vi "Lights and Music.vi"() -> ()   [LabVIEW 2013, in "LVH-Hue.lvlib"]
uses:
  LVH-Hue.lvlib
  <vilib>/sound2/lvsound2.llb/Sampling Mode.ctl
  Private/Type Defs/HSB.ctl
  <vilib>/sound2/lvsound2.llb/Sound File Info (path).vi
  <vilib>/sound2/lvsound2.llb/Sound File Read Open.vi
  <vilib>/sound2/lvsound2.llb/Sound File Read (DBL).vi
  <vilib>/measure/matone.llb/Extract Single Tone Information 1 Chan.vi
  Private/Set Light HSB By ID.vi
  <vilib>/sound2/lvsound2.llb/Sound Output Write (DBL Single).vi
  <vilib>/measure/NI_MAPro.lvlib
panel:
  in  "Hostname / IP":string="192.168.1.3"
  in  "Username":string="newdeveloper"
  in  "Lower Cut-Off":dbl=50.0
  out "Amp":dbl(graph)=0.00013614008667128265
  out "Freq":dbl(graph)=34.77410975578877
  out "detected frequency":dbl=34.77410975578877 format="%.2p"
  out "detected amplitude":dbl=0.00013614008667128265 format="%.2p"
  in  "Number of Samples/Iteration":i32=3500
  in  "Device ID":u32
  in  "Stop":bool
  out "Current Iteration":i32=32
  out "Raw Data":waveform(dbl)(graph)={"t0"=timestamp(1.8140589569160999 s since 1904-01-01), "dt"=2.2675736961451248e-05, "Y"=array[2500 elements]}
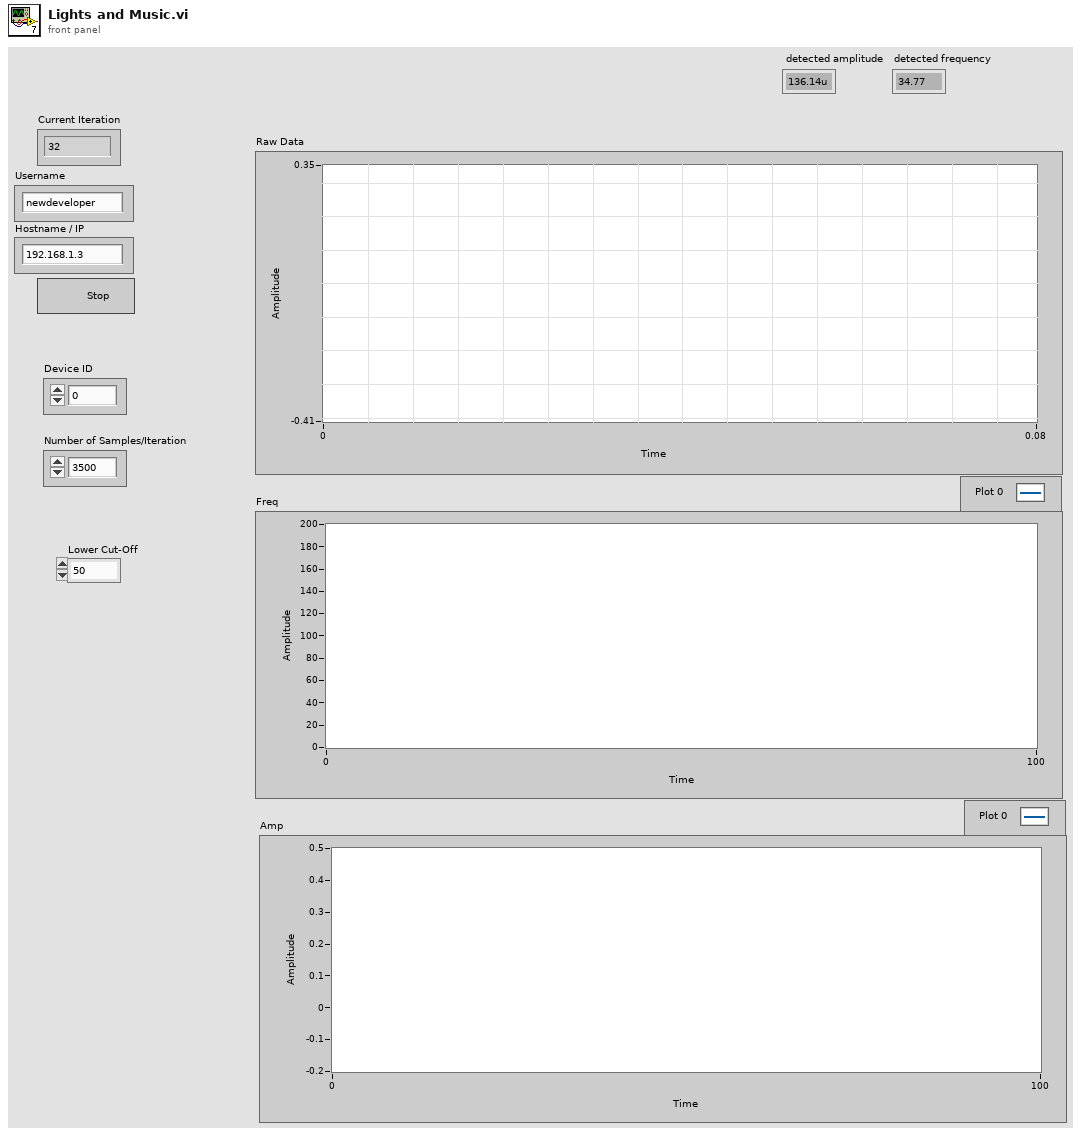
[diagram p1: front panel]
types:
  T1 = typedef "Sampling Mode.ctl" = i32
  T2 = typedef "Sound Data Format.ctl" = cluster{"sample rate (S/s)":dbl, "number of channels":i32, "bits per sample":i32}
  T3 = typedef "Sound File Refnum.ctl" = refnum<file>
  T4 = typedef "LVH-Hue.lvlib/Hue Ref.ctl" = cluster{"HTTP Session":T5, "Base URL":string, "Lights":T6[]}
  T5 = typedef "LabVIEWHTTPClient.lvlib/ClientHandle.ctl" = refnum<k1>
  T6 = typedef "LVH-Hue.lvlib/Light.ctl" = cluster{"ID":i32, "Name":string}
  T7 = typedef "Sound Output Task ID.ctl" = u32
  T8 = typedef "LVH-Hue.lvlib/HSB.ctl" = cluster{"Hue":u16, "Saturation":u8, "Brightness":u8}
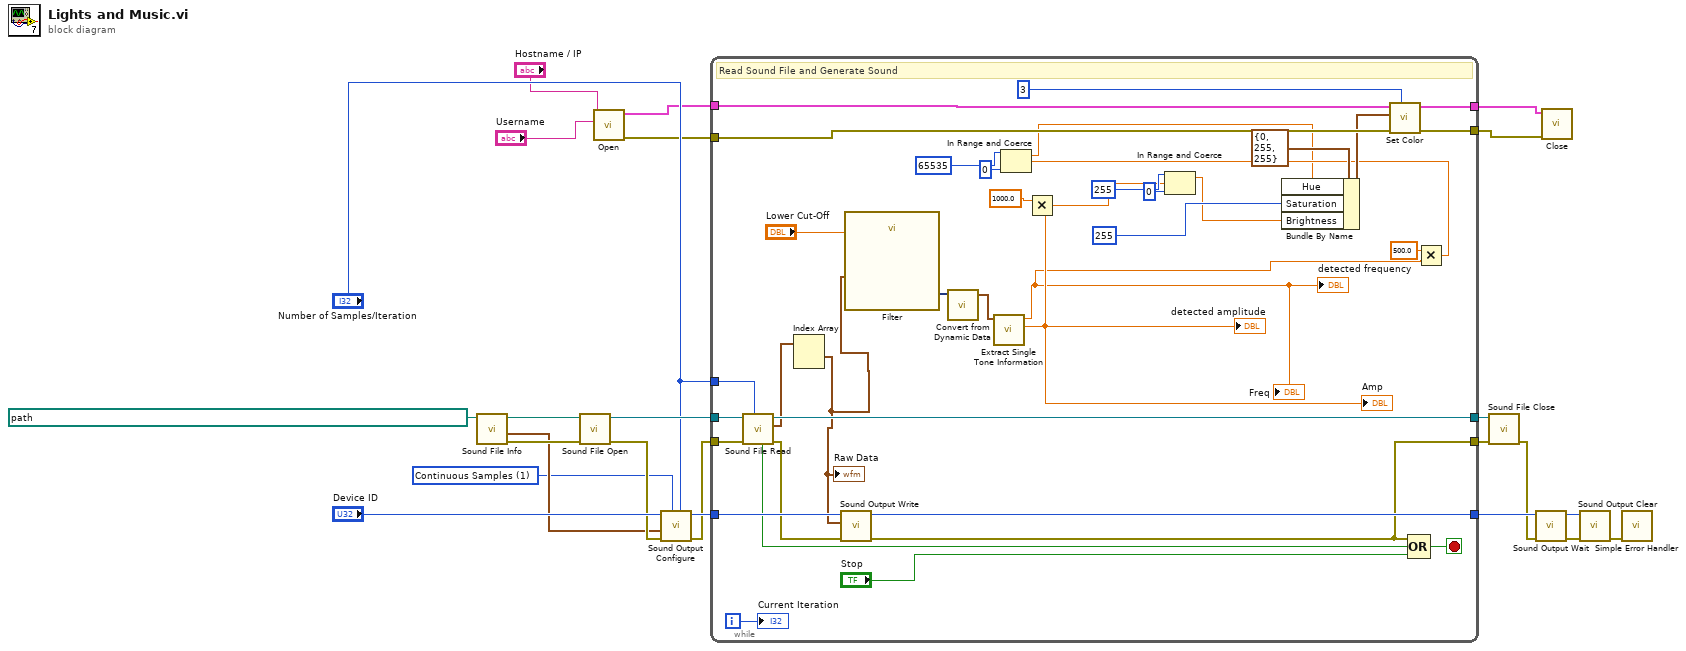
[diagram p0: block diagram]
diagram:
  w9 = T1 1 items=["Finite Samples", "Continuous Samples"] ("sample mode")
  n1 = call-poly <vilib>:"Sound File Info.vi"("path"=path "C:/Users/samkristoff/Downloads/Gotan Project - Lunático - 07 - Tango Canción.wav") -> ("error out"=w19:errorcluster, "sound format"=w11:T2, "path out"=w12:path)  [unwired: 7 in, 1 out]
  n2 = call-poly <vilib>:"Sound File Open.vi"("error in (no error)"=w19, "path"=w12) -> ("error out"=w18:errorcluster, "sound file refnum"=w20:T3)  [unwired: 8 in]
  n3 = call "Open.vi"("Username"="Username", "Hostname / IP"="Hostname / IP") -> ("Error Out"=w5:errorcluster, "Hue Config"=w6:T4)  [unwired: 8 in]
  n4 = call <vilib>:"Sound Output Configure.vi"("number of samples/ch"="Number of Samples/Iteration", "sample mode"=w9, "error in (no error)"=w18, "sound format"=w11, "device ID"="Device ID") -> ("error out"=w17:errorcluster, "task ID"=w24:T7)  [unwired: 5 in]
  n5 = while {
    tunnel: "Number of Samples/Iteration" -> [w51]
    tunnel: w20 -> [w59]
    tunnel: [w57] -> w22
    tunnel: w17 -> [w60]
    tunnel: [w50] -> w21
    tunnel: w24 -> [w56]
    tunnel: [w61] -> w15
    tunnel: w6 -> [w45]
    tunnel: w5 -> [w44]
    tunnel: [w39] -> w2
    tunnel: [w38] -> w1
    i -> [w58]
    stop <- w52 stop-if-true
    # "Read Sound File and Generate Sound"
    n6 = call-poly <vilib>:"Sound File Read.vi"("number of samples/ch (-1: all)"=w51, "error in (no error)"=w60, "sound file refnum"=w59) -> ("error out"=w55:errorcluster, "data"=w34:waveform(dbl)[], "sound file refnum out"=w57:T3, "end of file?"=w53:bool)  [unwired: 4 in, 1 out]
    n7 = Index Array(array=w34) -> (element #1=w33:waveform(dbl))  [unwired: 2 in, 1 out]
    "Raw Data" <- w33
    n8 = call-poly <vilib>:"Sound Output Write.vi"("error in (no error)"=w55, "data"=w33, "task ID"=w56) -> ("error out"=w50:errorcluster, "task ID out"=w61:T7)  [unwired: 7 in]
    n9 = call "Filter"("Lower Cut-Off"="Lower Cut-Off", "Signal"=w33) -> ("Filtered Signal"=w48:dynamicdata)  [unwired: 8 in, 1 out]
    n10 = call "Convert from Dynamic Data"("Dynamic Data Type"=w48) -> ("Waveform"=w47:waveform(dbl))  [unwired: 3 in]
    n11 = call-poly <vilib>:"Extract Single Tone Information.vi"("time signal in"=w47) -> ("detected amplitude"=w43:dbl, "detected frequency"=w36:dbl)  [unwired: 5 in, 4 out]
    "detected amplitude" <- w43
    "detected frequency" <- w36
    "Freq" <- w36
    "Amp" <- w43
    n12 = Multiply(x=1000.0, y=w43) -> (x*y=w26:dbl)
    n13 = In Range and Coerce(upper limit=u16 255 ("Hue"), x=w26, lower limit=u16 0) -> (coerced(x)=w25:dbl)  [unwired: 1 out]
    n14 = Compound Arithmetic op=OR(w50, w53, "Stop") -> (w52:bool)
    n15 = Multiply(x=500.0, y=w36) -> (x*y=w30:dbl)
    n16 = In Range and Coerce(upper limit=u16 65535 ("Hue"), x=w30, lower limit=u16 0) -> (coerced(x)=w29:dbl)  [unwired: 1 out]
    n17 = Bundle By Name(cluster=T8 {"Hue"=0, "Saturation"=255, "Brightness"=255} ("HSB"), "Hue"=w29, "Saturation"=u8 255, "Brightness"=w25) -> (w35:T8)
    n18 = call-poly "Set Color.vi"("ID"=u8 3, "Error In"=w44, "HSB"=w35, "Hue Config"=w45) -> ("Error Out"=w39:errorcluster, "Hue Config"=w38:T4)  [unwired: 6 in]
    "Current Iteration" <- w58
  }
  n19 = call <vilib>:"Sound File Close.vi"("error in (no error)"=w21, "sound file refnum"=w22) -> ("error out"=w14:errorcluster)  [unwired: 9 in]
  n20 = call <vilib>:"Sound Output Wait.vi"("error in (no error)"=w14, "task ID"=w15) -> ("error out"=w13:errorcluster, "task ID out"=w16:T7)  [unwired: 8 in]
  n21 = call "Close.vi"("Error In"=w2, "Hue Config"=w1) -> ()  [unwired: 9 in, 1 out]
  n22 = call <vilib>:"Sound Output Clear.vi"("error in (no error)"=w13, "task ID"=w16) -> ("error out"=w8:errorcluster)  [unwired: 9 in]
  n23 = call <vilib>:"Simple Error Handler.vi"("error in (no error)"=w8) -> ()  [unwired: 4 in, 5 out]
